vi "test_hwtiming.vi"(8 "error in":errorcluster) -> (0 "error out":errorcluster)   [LabVIEW 2012]
uses:
  <vilib>/DAQmx/write.llb/DAQmx Write (Digital Wfm 1Chan NSamp).vi
  <vilib>/Waveform/DWDTOps.llb/Digital Pattern Generator (Single Value).vi
  <vilib>/DAQmx/create/channels.llb/DAQmx Create Channel (DO-Digital Output).vi
  <vilib>/Waveform/DWDTOps.llb/DWDT Append Digital Samples.vi
  <vilib>/Waveform/DWDTOps.llb/DWDT Digital Size.vi
  <vilib>/DAQmx/configure/timing.llb/DAQmx Timing (Sample Clock).vi
  <vilib>/Waveform/DWDTOps.llb/DWDT Uncompress Digital.vi
  <vilib>/DAQmx/miscellaneous.llb/DAQmx Fill In Error Info.vi
  <resource>/objmgr/daqmx.rc
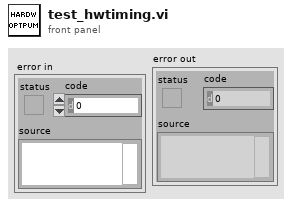
[diagram p1: front panel]
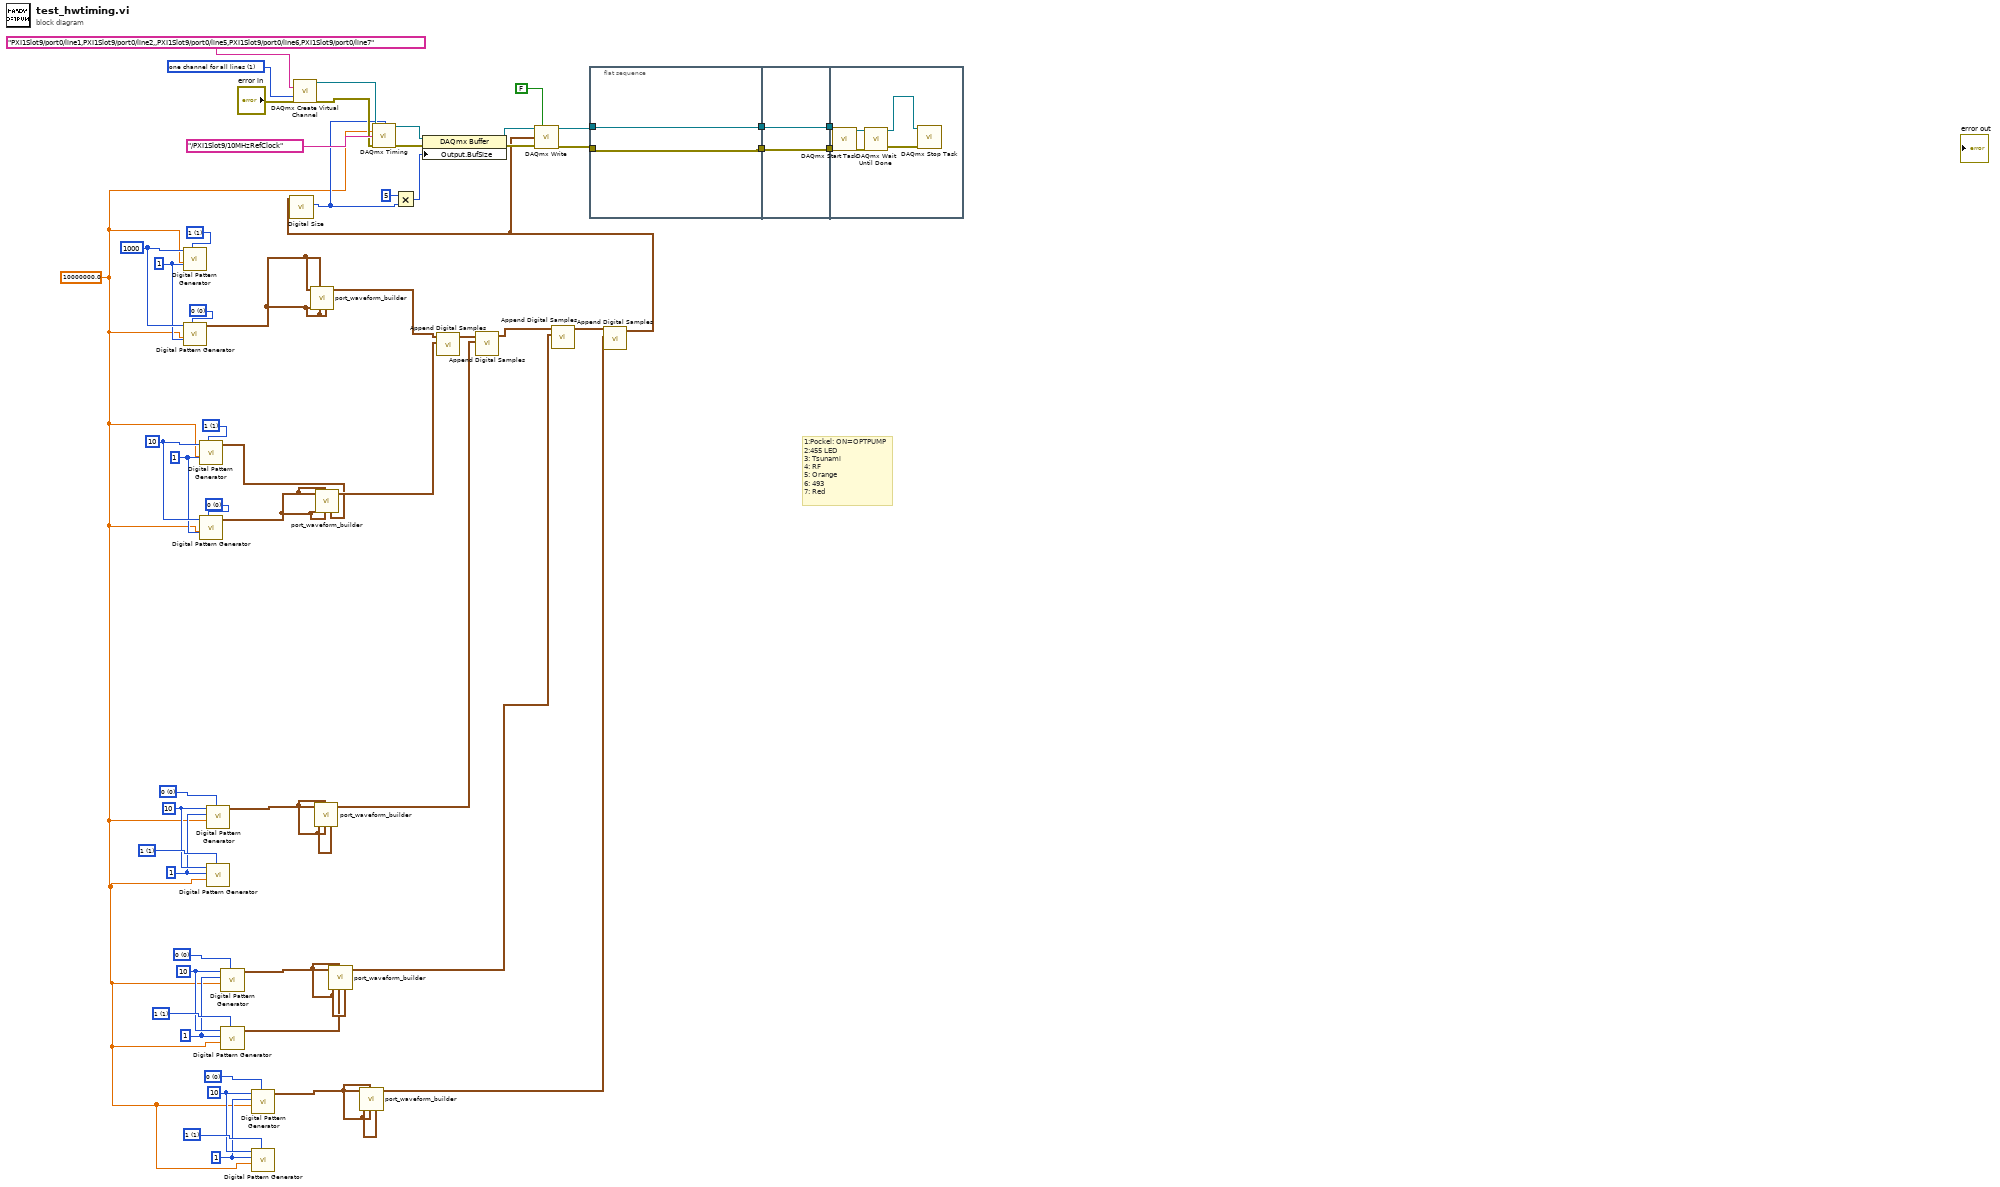
[diagram p0: block diagram]
diagram:
  w9 = u8 0 items=["0", "1", "Z", "L", "H", "X", "T", "V"] ("value")
  w7 = u32 1 ("number of signals")
  w8 = u32 10 ("number of samples")
  w10 = u8 1 items=["0", "1", "Z", "L", "H", "X", "T", "V"] ("value")
  w17 = u8 0 items=["0", "1", "Z", "L", "H", "X", "T", "V"] ("value")
  w15 = u32 1 ("number of signals")
  w16 = u32 10 ("number of samples")
  w18 = u8 1 items=["0", "1", "Z", "L", "H", "X", "T", "V"] ("value")
  w31 = u8 0 items=["0", "1", "Z", "L", "H", "X", "T", "V"] ("value")
  w29 = u32 1 ("number of signals")
  w30 = u32 10 ("number of samples")
  w32 = u8 1 items=["0", "1", "Z", "L", "H", "X", "T", "V"] ("value")
  w38 = u8 0 items=["0", "1", "Z", "L", "H", "X", "T", "V"] ("value")
  w36 = u32 1 ("number of signals")
  w37 = u32 10 ("number of samples")
  w39 = u8 1 items=["0", "1", "Z", "L", "H", "X", "T", "V"] ("value")
  w44 = u8 0 items=["0", "1", "Z", "L", "H", "X", "T", "V"] ("value")
  w42 = u32 1 ("number of signals")
  w43 = u32 1000 ("number of samples")
  w45 = u8 1 items=["0", "1", "Z", "L", "H", "X", "T", "V"] ("value")
  w50 = 1 items=["one channel for each line", "one channel for all lines"] ("line grouping")
  w5 = 10000000.0 ("rate")
  # "1:Pockel: ON=OPTPUMP\n2:455 LED\n3: Tsunami\n4: RF\n5: Orange\n6: 493\n7: Red"
  n1 = call-poly <vilib>:"Digital Pattern Generator.vi"("value"=w45, "sample rate"=w5, "number of signals"=w42, "number of samples"=w43) -> ()  [unwired: 6 in, 2 out]
  n2 = call-poly <vilib>:"Digital Pattern Generator.vi"("value"=w44, "sample rate"=w5, "number of signals"=w42, "number of samples"=w43) -> ("digital waveform"=w22:digitalwaveform)  [unwired: 6 in, 1 out]
  n3 = call-poly <vilib>:"Digital Pattern Generator.vi"("value"=w39, "sample rate"=w5, "number of signals"=w36, "number of samples"=w37) -> ("digital waveform"=w19:digitalwaveform)  [unwired: 6 in, 1 out]
  n4 = call-poly <vilib>:"Digital Pattern Generator.vi"("value"=w38, "sample rate"=w5, "number of signals"=w36, "number of samples"=w37) -> ("digital waveform"=w1:digitalwaveform)  [unwired: 6 in, 1 out]
  n5 = call-poly <vilib>:"Digital Pattern Generator.vi"("value"=w31, "sample rate"=w5, "number of signals"=w29, "number of samples"=w30) -> ("digital waveform"=w20:digitalwaveform)  [unwired: 6 in, 1 out]
  n6 = call-poly <vilib>:"Digital Pattern Generator.vi"("value"=w32, "sample rate"=w5, "number of signals"=w29, "number of samples"=w30) -> ()  [unwired: 6 in, 2 out]
  n7 = call-poly <vilib>:"Digital Pattern Generator.vi"("value"=w17, "sample rate"=w5, "number of signals"=w15, "number of samples"=w16) -> ("digital waveform"=w14:digitalwaveform)  [unwired: 6 in, 1 out]
  n8 = call-poly <vilib>:"Digital Pattern Generator.vi"("value"=w18, "sample rate"=w5, "number of signals"=w15, "number of samples"=w16) -> ("digital waveform"=w13:digitalwaveform)  [unwired: 6 in, 1 out]
  n9 = call-poly <vilib>:"Digital Pattern Generator.vi"("value"=w9, "sample rate"=w5, "number of signals"=w7, "number of samples"=w8) -> ("digital waveform"=w6:digitalwaveform)  [unwired: 6 in, 1 out]
  n10 = call-poly <vilib>:"Digital Pattern Generator.vi"("value"=w10, "sample rate"=w5, "number of signals"=w7, "number of samples"=w8) -> ()  [unwired: 6 in, 2 out]
  n11 = call-poly <vilib>:"DAQmx Create Virtual Channel.vi"("lines"=tag "PXI1Slot9/port0/line1,PXI1Slot9/port0/line2,,PXI1Slot9/port0/line5,PXI1Slot9/port0/line6,PXI1Slot9/port0/line7", "line grouping"=w50, "error in"="error in") -> ("task out"=w51:refnum<k21>, "error out"=w48:errorcluster)  [unwired: 11 in]
  n12 = call "port_waveform_builder.vi"("Line 7"=w22, "Line 6"=w22, "Line 1"=w22, "Line 5"=w22, "Line 2"=w22) -> ("digital waveform out"=w35:digitalwaveform)  [unwired: 6 in]
  n13 = call "port_waveform_builder.vi"("Line 7"=w20, "Line 6"=w20, "Line 1"=w20, "Line 5"=w20, "Line 2"=w20) -> ("digital waveform out"=w21:digitalwaveform)  [unwired: 6 in]
  n14 = call "port_waveform_builder.vi"("Line 7"=w19, "Line 6"=w1, "Line 1"=w1, "Line 5"=w1, "Line 2"=w1) -> ("digital waveform out"=w34:digitalwaveform)  [unwired: 6 in]
  n15 = call "port_waveform_builder.vi"("Line 7"=w14, "Line 6"=w13, "Line 1"=w14, "Line 5"=w14, "Line 2"=w14) -> ("digital waveform out"=w11:digitalwaveform)  [unwired: 6 in]
  n16 = call "port_waveform_builder.vi"("Line 7"=w6, "Line 6"=w6, "Line 1"=w6, "Line 5"=w6, "Line 2"=w6) -> ("digital waveform out"=w2:digitalwaveform)  [unwired: 6 in]
  n17 = call-poly <vilib>:"Append Digital Samples.vi"("digital waveform B"=w34, "digital waveform A"=w35) -> ("digital waveform out"=w33:digitalwaveform)  [unwired: 8 in, 1 out]
  n18 = call-poly <vilib>:"Append Digital Samples.vi"("digital waveform B"=w21, "digital waveform A"=w33) -> ("digital waveform out"=w12:digitalwaveform)  [unwired: 8 in, 1 out]
  n19 = call-poly <vilib>:"Append Digital Samples.vi"("digital waveform B"=w11, "digital waveform A"=w12) -> ("digital waveform out"=w4:digitalwaveform)  [unwired: 8 in, 1 out]
  n20 = flat-sequence {
    tunnel: w46 -> [w58]
    tunnel: w52 -> [w59]
    tunnel: [w59] -> w28
    tunnel: [w58] -> w25
    tunnel: w28 -> [w61]
    tunnel: [w61] -> w27
    tunnel: [w60] -> w26
    tunnel: w25 -> [w60]
    tunnel: w27 -> [w67]
    tunnel: w26 -> [w66]
    frame #0 {
    }
    frame #1 {
    }
    frame #2 {
      n21 = call <vilib>:"DAQmx Start Task.vi"("task/channels in"=w67, "error in"=w66) -> ("task out"=w64:refnum<k21>, "error out"=w65:errorcluster)  [unwired: 12 in]
      n22 = call <vilib>:"DAQmx Wait Until Done.vi"("task/channels in"=w64, "error in"=w65) -> ("task out"=w62:refnum<k21>, "error out"=w63:errorcluster)  [unwired: 12 in]
      n23 = call <vilib>:"DAQmx Stop Task.vi"("task/channels in"=w62, "error in"=w63) -> ()  [unwired: 12 in, 2 out]
    }
  }
  n24 = call-poly <vilib>:"Append Digital Samples.vi"("digital waveform B"=w2, "digital waveform A"=w4) -> ("digital waveform out"=w3:digitalwaveform)  [unwired: 8 in, 1 out]
  n25 = call-poly <vilib>:"Digital Size.vi"("digital waveform in"=w3) -> ("number of samples"=w23:i32)  [unwired: 7 in, 3 out]
  n26 = call-poly <vilib>:"DAQmx Timing.vi"("task/channels in"=w51, "samples per channel"=w23, "rate"=w5, "source"=tag "/PXI1Slot9/10MHzRefClock", "error in"=w48) -> ("task out"=w56:refnum<k21>, "error out"=w55:errorcluster)  [unwired: 9 in]
  n27 = Multiply(x=5, y=w23) -> (x*y=w24:i32)
  n28 = property class="DAQmx Buffer"(reference=w56, error in=w55, "Output.BufSize"=w24) -> (reference out=w53:refnum<k21>, error out=w47:errorcluster)
  n29 = call-poly <vilib>:"DAQmx Write.vi"("task/channels in"=w53, "auto start"=FALSE, "data"=w3, "error in"=w47) -> ("task out"=w52:refnum<k21>, "error out"=w46:errorcluster)  [unwired: 9 in, 1 out]
